vi "TimeCounter.vi"(8 "error in (no error)":errorcluster, 9 "Monh of Year in":u32, 10 "Day of Year in":u32, 11 "Daytime in":u32) -> (0 "error out":errorcluster, 1 "Monh of Year out":u32, 2 "Day of Year out":u32, 3 "Daytime out":u32)   [LabVIEW 2017]
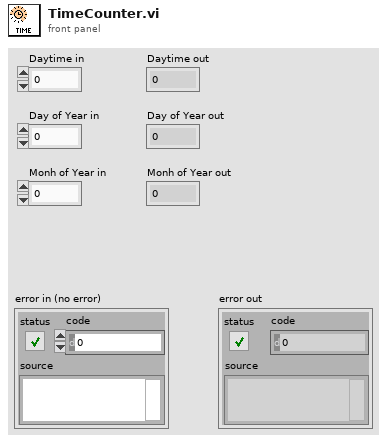
[diagram p1: front panel]
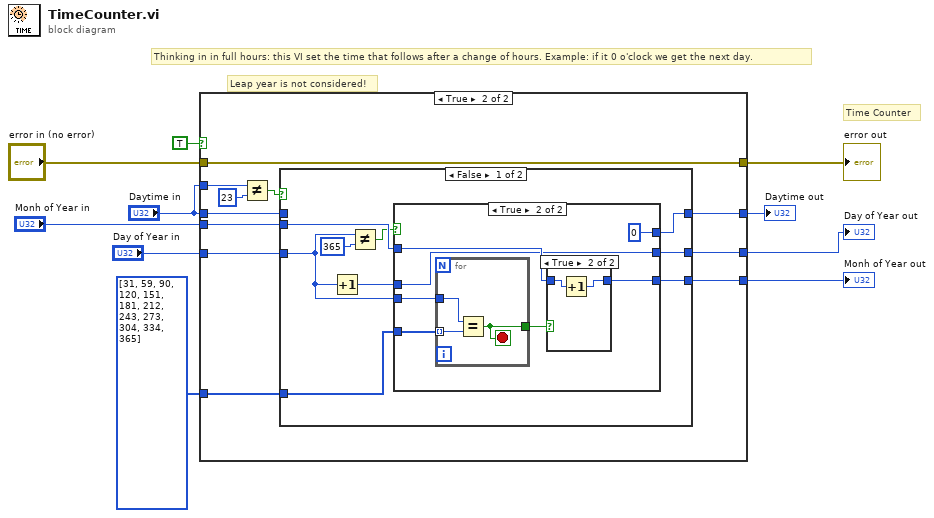
[diagram p0: block diagram]
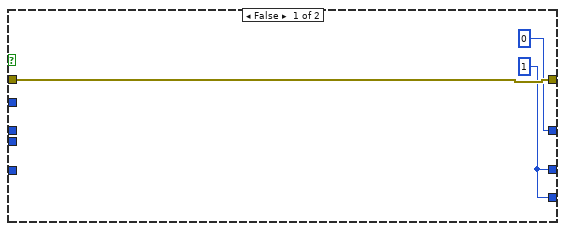
[diagram p2: hidden frame]
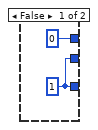
[diagram p3: hidden frame]
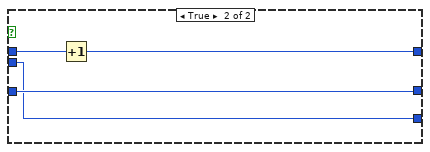
[diagram p5: hidden frame]
diagram:
  # "Thinking in in full hours: this VI set the time that follows after a change of hours. Example: if it 0 o'clock we get the next day."
  # "Leap year is not considered!"
  # "Time Counter"
  n1 = case shown="True" TRUE {
    tunnel: [w12 w24] -> w9
    tunnel: "Day of Year in" -> [_ w23]
    tunnel: [w13 w22] -> w8
    tunnel: "error in (no error)" -> [w13 w22]
    tunnel: [w12 w21] -> w7
    tunnel: "Monh of Year in" -> [_ w20]
    tunnel: u32[] [31, 59, 90, 120, 151, 181, 212, 243, 273, 304, 334, 365] -> [_ w19]
    tunnel: "Daytime in" -> [_ w16]
    tunnel: [u32 0 ("Timer-Wert (ms)") w14] -> w4
    tunnel: "Daytime in" -> [_ w15]
    frame False {
      w12 = u32 1 ("Timer-Wert (ms)")
    }
    frame True {
      n2 = Not Equal?(x=w16, y=u32 23) -> (x != y?=w17:bool)
      n3 = case shown="False" w17 {
        tunnel: [w25 w52] -> w24
        tunnel: w23 -> [w26 w52]
        tunnel: [w33 w51] -> w21
        tunnel: w20 -> [w31 w51]
        tunnel: w19 -> [w32 _]
        tunnel: w15 -> [_ w50]
        tunnel: [w30 w49] -> w14
        frame False {
          n4 = Increment(x=w26) -> (x+1=w27:u32)
          n5 = Not Equal?(x=w26, y=u32 365) -> (x != y?=w28:bool)
          n6 = case shown="True" w28 {
            tunnel: [w35 w36] -> w25
            tunnel: [w35 w41] -> w33
            tunnel: w32 -> [_ w40]
            tunnel: w31 -> [_ w39]
            tunnel: w26 -> [_ w38]
            tunnel: [u32 0 ("Timer-Wert (ms)") u32 0] -> w30
            tunnel: w27 -> [_ w36]
            frame False {
              w35 = u32 1 ("Timer-Wert (ms)")
            }
            frame True {
              n7 = for {
                tunnel: w40 -> [w47] mode=indexing
                tunnel: w38 -> [w48]
                tunnel: [w46] -> w42
                stop <- w46 stop-if-true
                n8 = Equal?(x=w48, y=w47) -> (x = y?=w46:bool)
              }
              n9 = case shown="True" w42 {
                tunnel: w39 -> [w43 w45]
                tunnel: [w43 w44] -> w41
                frame False {
                }
                frame True {
                  n10 = Increment(x=w45) -> (x+1=w44:u32)
                }
              }
            }
          }
        }
        frame True {
          n11 = Increment(x=w50) -> (x+1=w49:u32)
        }
      }
    }
  }
  "Monh of Year out" <- w7
  "Day of Year out" <- w9
  "Daytime out" <- w4
  "error out" <- w8
